vi "存储Data至数据库.vi"(8 "error in (no error)":errorcluster caption="错误输入（无错误）", 11 "DB Con":refnum<class "Connection.lvclass">) -> (0 "error out":errorcluster caption="错误输出", 3 "DB Con 2":refnum<class "Connection.lvclass">)   [LabVIEW 2018]
uses:
  <vilib>/drjdpowell/SQLite Library/SQL Connection/Connection.lvclass
  <vilib>/drjdpowell/SQLite Library/SQL Statement/SQL Statement.lvclass/SQL Statement.ctl
  <vilib>/drjdpowell/SQLite Library/SQL Statement/Bind Timestamp (Julian Day).vi
  <vilib>/drjdpowell/SQLite Library/SQL Statement/Bind Real.vi
  <vilib>/JDP Science/JDP Science Common Utilities/Trim Whitespace__JDP.vi
  <vilib>/drjdpowell/SQLite Library/SQL Statement/Step.vi
  <vilib>/drjdpowell/SQLite Library/SQL Statement/Error Message.vi
  <vilib>/drjdpowell/SQLite Library/SQL Statement/SQL Statement.lvclass
  <vilib>/drjdpowell/SQLite Library/Transaction Helpers/Transaction.lvlib
  <vilib>/drjdpowell/SQLite Library/SQLite.lvlib
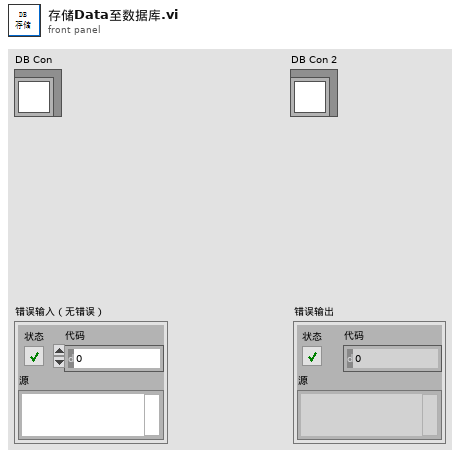
[diagram p1: front panel]
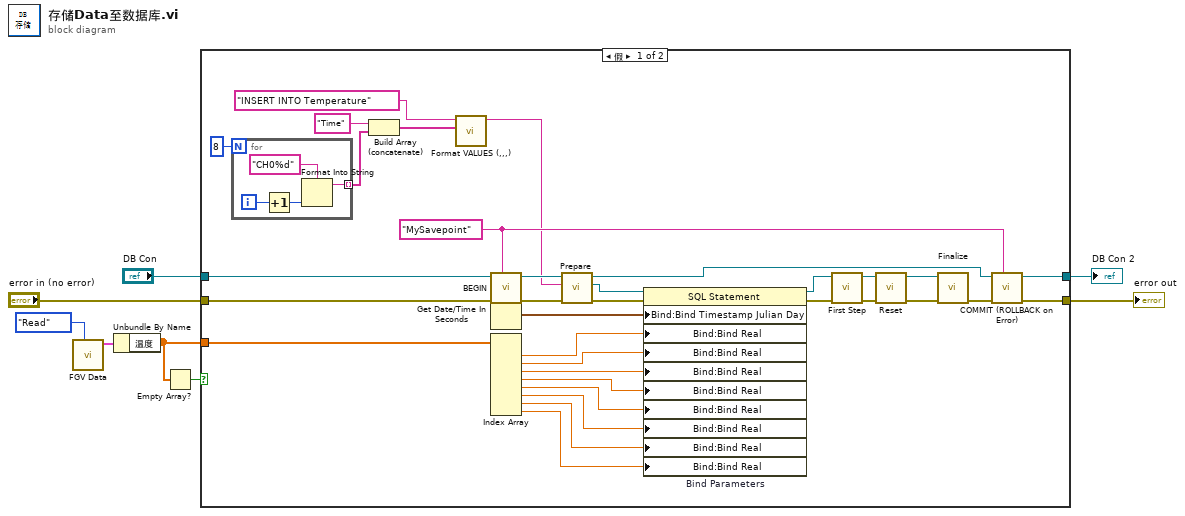
[diagram p0: block diagram]
diagram:
  n1 = call "FGV Data.vi"("Action"=enum16{"Initial", "Read", "Write"}."Read") -> ("Data OUT"=w7:cluster{"Con?":bool, "温度":dbl[]})  [unwired: 9 in, 1 out]
  n2 = Unbundle By Name(w7) -> ("温度"=w2:dbl[])
  n3 = Empty Array?(array=w2) -> (empty?=w1:bool)
  n4 = case shown="假" w1 {
    tunnel: [w18 w46] -> w6
    tunnel: "DB Con" -> [w12 w47]
    tunnel: "error in (no error)" -> [w11 w46]
    tunnel: w2 -> [w10 _]
    tunnel: [w9 w47] -> w3
    frame False {
      w38 = "MySavepoint" ("Savepoint name")
      n5 = for {
        N: 8 -> [_]
        tunnel: [w42] -> w16 mode=indexing
        i -> [w45]
        n6 = Increment(x=w45) -> (x+1=w44:i32)
        n7 = Format Into String(format string="CH0%d" ("格式字符串"), w44) -> (resulting string=w42:string)  [unwired: 2 in, 1 out]
      }
      n8 = Build Array (concatenate)("Time", w16) -> (w15:string[])
      n9 = call <vilib>:"Format VALUES (,,,).vi"("Column Names"=w15, "partial SQL"="INSERT INTO Temperature") -> ("SQL"=w13:string)  [unwired: 9 in]
      n10 = call <vilib>:"BEGIN.vi"("Savepoint name"=w38, "error in (no error)"=w11, "SQLite Connection in"=w12) -> ("error out"=w37:errorcluster, "SQLite Connection"=w36:refnum<class "Connection.lvclass">)  [unwired: 7 in]
      n11 = Get Date/Time In Seconds() -> (seconds since 1Jan1904=w27:timestamp)
      n12 = Index Array(array=w10) -> (element #1=w26:dbl, element #2=w25:dbl, element #3=w24:dbl, element #4=w23:dbl, element #5=w22:dbl, element #6=w21:dbl, element #7=w20:dbl, element #8=w19:dbl)  [unwired: 8 in]
      n13 = call <vilib>:"Prepare.vi"("error in (no error)"=w37, "SQL"=w13, "SQLite Connection in"=w36) -> ("error out"=w33:errorcluster, "SQL Statement"=w32:refnum<class "SQL Statement.lvclass">, "SQLite Connection"=w39:refnum<class "Connection.lvclass">)  [unwired: 4 in, 2 out]
      n14 = property on="Bind Parameters" class="SQL Statement"(reference=w32, error in=w33, "Bind:Bind Timestamp Julian Day"=w27, "Bind:Bind Real"=w26, "Bind:Bind Real"=w25, "Bind:Bind Real"=w24, "Bind:Bind Real"=w23, "Bind:Bind Real"=w22, "Bind:Bind Real"=w21, "Bind:Bind Real"=w20, "Bind:Bind Real"=w19) -> (reference out=w31:refnum<class "SQL Statement.lvclass">, error out=w30:errorcluster)
      n15 = call <vilib>:"First Step.vi"("error in (no error)"=w30, "SQL Statement in"=w31) -> ("error out"=w29:errorcluster, "SQL Statement"=w28:refnum<class "SQL Statement.lvclass">)  [unwired: 7 in, 1 out]
      n16 = call <vilib>:"Reset.vi"("error in (no error)"=w29, "SQL Statement in"=w28) -> ("error out"=w35:errorcluster, "SQL Statement"=w34:refnum<class "SQL Statement.lvclass">)  [unwired: 8 in]
      n17 = call <vilib>:"Finalize.vi"("error in (no error)"=w35, "SQL Statement in"=w34) -> ("error out"=w40:errorcluster)  [unwired: 9 in]
      n18 = call <vilib>:"COMMIT (ROLLBACK on Error).vi"("Savepoint name"=w38, "error in (no error)"=w40, "SQLite Connection in"=w39) -> ("error out"=w18:errorcluster, "SQLite Connection"=w9:refnum<class "Connection.lvclass">)  [unwired: 7 in]
    }
    frame True {
    }
  }
  "error out" <- w6
  "DB Con 2" <- w3
